vi "Set UAV Marker Position.vi"(8 "error in (no error)":errorcluster, 10 "lon":dbl=150.8617687 format="%#_13g", 11 "lat":dbl=-31.1105459 format="%#_13g") -> (0 "error out":errorcluster)   [LabVIEW 2014]
uses:
  C:/Robotic Systems/Products/AgFalcon/Software/Ground Station/Data/Mapping DLL/GMap.NET.Core.dll
  Data/Mapping DLL/GMap.NET.Core.dll
  C:/Robotic Systems/Products/AgFalcon/Software/Ground Station/Data/Mapping DLL/GMap.NET.WindowsForms.dll
  Data/Mapping DLL/GMap.NET.WindowsForms.dll
  Reference/SubVI/GMap DLL Refernce.vi
  Reference/SubVI/Main Map Control Refernce.vi
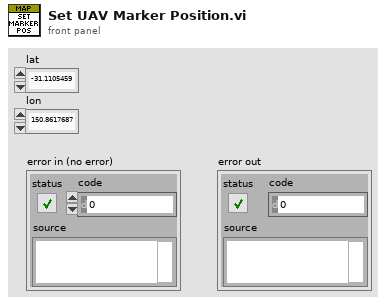
[diagram p1: front panel]
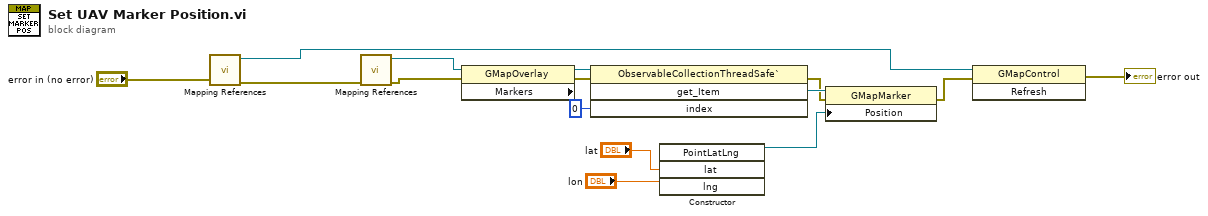
[diagram p0: block diagram]
diagram:
  n1 = call-poly "Mapping References.vi"("Error In"="error in (no error)") -> ("Error Out"=w2:errorcluster, "GMap DLL Reference"=w5:refnum<k24>)  [unwired: 9 in]
  n2 = call-poly "Mapping References.vi"("Error In"=w2) -> ("Error Out"=w3:errorcluster, "Main Map Reference"=w4:refnum<k24>)  [unwired: 9 in]
  n3 = property class="GMapOverlay"(reference=w4, error in=w3) -> (error out=w6:errorcluster, "Markers"=w12:refnum<k24>)  [unwired: 1 out]
  n4 = invoke class="ObservableCollectionThreadSafe`" method="get_Item"(reference=w12, error in=w6, "index"=0) -> (error out=w7:errorcluster, "get_Item"=w10:refnum<k24>)  [unwired: 1 in, 2 out]
  n5 = constructor class="PointLatLng"("lat"="lat", "lng"="lon") -> (reference out=w9:refnum<k24>)  [unwired: 3 in, 4 out]
  n6 = property class="GMapMarker"(reference=w10, error in=w7, "Position"=w9) -> (error out=w8:errorcluster)  [unwired: 1 out]
  n7 = invoke class="GMapControl" method="Refresh"(reference=w5, error in=w8) -> (error out=→"error out":errorcluster)  [unwired: 1 in, 2 out]
